vi "Trace Level for Error.vi"(8 "error in (no error)":errorcluster, 10 "Requested Trace Level":T1, 11 "System Actor in":refnum<class "System Actor.lvclass">) -> (0 "error out":errorcluster, 2 "Trace Level for Error":T1, 3 "System Actor out":refnum<class "System Actor.lvclass">)   [LabVIEW 2014, in "Robot Actor Framework.lvlib" / "System Actor.lvlib" / "System Actor.lvclass"]
uses:
  System Actor.lvclass
  Trace/Trace Class/Trace Levels.ctl
  Trace/Trace Class/Trace.lvclass
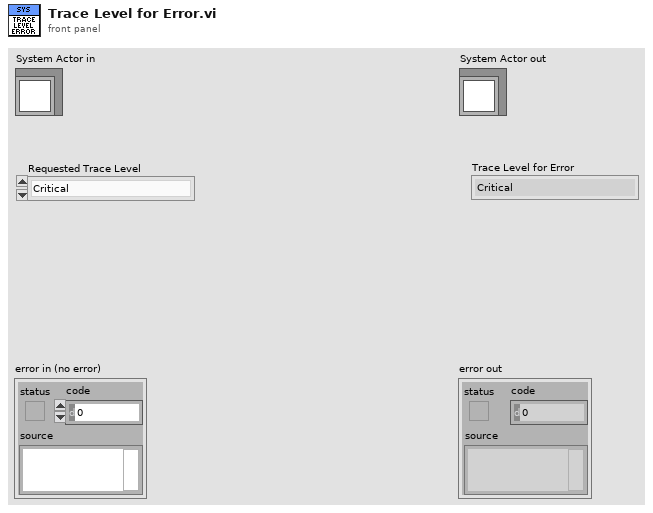
[diagram p1: front panel]
types:
  T1 = typedef "Robot Actor Framework.lvlib/Trace.lvlib/Trace.lvclass/Trace Levels.ctl" = enum16{"Critical", "Error", "Warning", "Informational", "Debug"}
  T2 = enum16{"Critical", "Error", "Warning", "Informational", "Debug"}
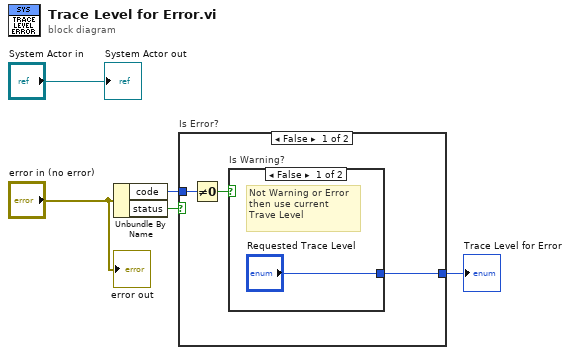
[diagram p0: block diagram]
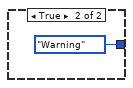
[diagram p2: hidden frame]
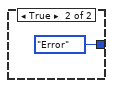
[diagram p3: hidden frame]
diagram:
  n1 = Unbundle By Name("error in (no error)") -> ("code"=w1:i32, "status"=w4:bool)
  n2 = case "Is Error?" shown="False" w4 {
    tunnel: [w7 T2."Error" ("Trace Level")] -> w3
    tunnel: w1 -> [w6 _]
    frame False {
      n3 = Not Equal To 0?(x=w6) -> (x != 0?=w8:bool)
      n4 = case "Is Warning?" shown="False" w8 {
        tunnel: ["Requested Trace Level" T2."Warning" ("Trace Level")] -> w7
        frame False {
          # "Not Warning or Error\nthen use current\nTrave Level"
        }
        frame True {
        }
      }
    }
    frame True {
    }
  }
  "Trace Level for Error" <- w3
  "error out" <- "error in (no error)"
  "System Actor out" <- "System Actor in"
